vi "Test Missing Libraries.vi"(8 "error in":errorcluster, 11 "My Computer":refnum<vi>) -> (0 "error out":errorcluster, 4 "Missing items from LabVIEW project":path[](array[path]), 5 "Pass":bool)   [LabVIEW 2020, in "Missing in Project Tests.lvlib"]
doc: "Tests to make sure all libraries defined in the project are saved to disk."
uses:
  Missing in Project Tests.lvlib
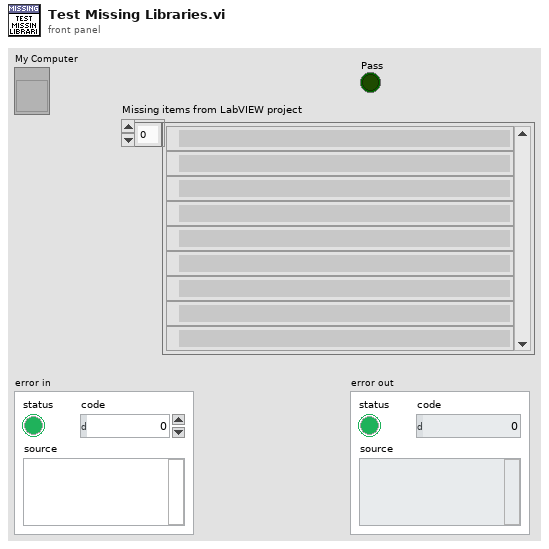
[diagram p1: front panel]
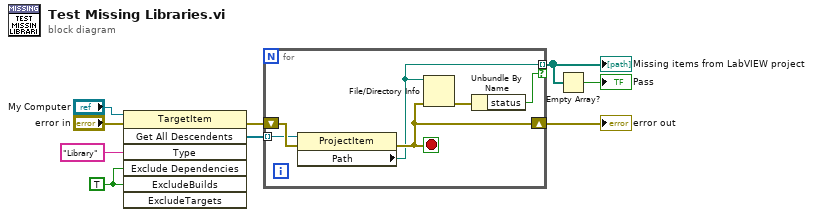
[diagram p0: block diagram]
diagram:
  w2 = TRUE ("ExcludeBuilds")
  n1 = invoke class="TargetItem" method="Get All Descendents"(reference="My Computer", error in="error in", "Type"="Library", "Exclude Dependencies"=w2, "ExcludeBuilds"=w2) -> (error out=w9:errorcluster, "All Descendents"=w5:refnum<vi>[])  [unwired: 2 in, 5 out]
  n2 = for {
    tunnel: w5 -> [w12] mode=indexing
    shift-right: [w13] -> w7
    shift-left: w9 -> [w14]
    tunnel: [w11] -> w3 mode=indexing if=w10
    stop <- w13 stop-if-true
    n3 = property class="ProjectItem"(reference=w12, error in=w14) -> (error out=w13:errorcluster, "Path"=w11:path)  [unwired: 1 out]
    n4 = File/Directory Info(path=w11, error in=w13) -> (error out=w15:errorcluster)  [unwired: 6 out]
    n5 = Unbundle By Name(w15) -> ("status"=w10:bool)
  }
  "Missing items from LabVIEW project" <- w3
  "error out" <- w7
  n6 = Empty Array?(array=w3) -> (empty?=→"Pass":bool)
